vi "Read Results from processing.vi"(8 "error in":errorcluster, 11 "LED runtime in":refnum<class "LED runtime.lvclass">) -> (0 "error out":errorcluster, 2 "Results from processing":T1, 3 "LED runtime out":refnum<class "LED runtime.lvclass">)   [LabVIEW 2013, in "LED runtime.lvclass"]
uses:
  LED runtime.lvclass
  configuration/result data indices.ctl
  LED runtime.lvclass/LED runtime.ctl
  configuration/LED configuration.lvclass
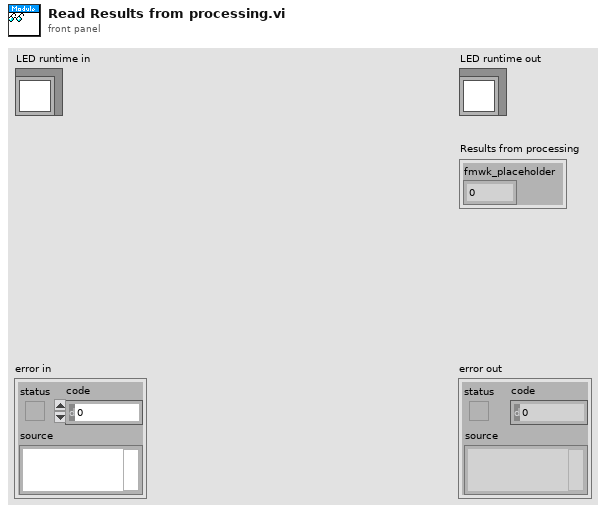
[diagram p1: front panel]
types:
  T1 = typedef "LED configuration.lvclass/result data indices.ctl" = cluster{"fmwk_placeholder":i32}
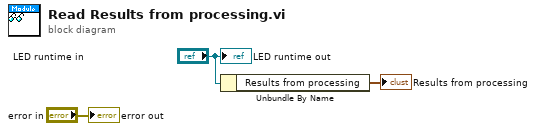
[diagram p0: block diagram]
diagram:
  n1 = Unbundle By Name("LED runtime in") -> ("Results from processing"=→"Results from processing":T1)
  "error out" <- "error in"
  "LED runtime out" <- "LED runtime in"
